vi "AudioStreamer.Globals.vi"() -> ()   [LabVIEW 2020]
uses:
  AudioStreamer.Config.ctl
panel:
  in  "config":T1
  out "triggered":bool
  out "running":bool
  out "last error":errorcluster
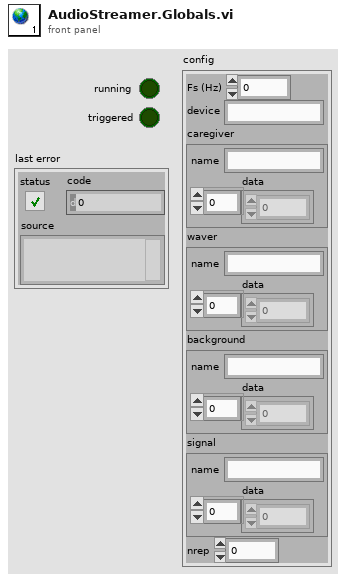
[diagram p1: front panel]
types:
  T1 = typedef "AudioStreamer.Config.ctl" = cluster{"Fs (Hz)":dbl, "device":string, "caregiver":cluster{"name":string, "data":dbl[]}, "waver":cluster{"name":string, "data":dbl[]}, "background":cluster{"name":string, "data":dbl[]}, "signal":cluster{"name":string, "data":dbl[]}, "nrep":i32}
diagram:
